vi "update全局.vi"() -> ()   [LabVIEW 2016, in "数据传输系统.lvlib"]
panel:
  in  "updateconfiguration":cluster{"IP地址":string, "端口号":i32}={"IP地址"="27.154.58.30", "端口号"=11234}
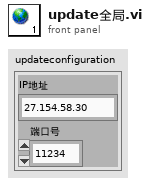
[diagram p1: front panel]
diagram:
